vi "Teleop.vi"(10 "Match Info":T1={"Autonomous Elapsed Seconds"=0.0, "TeleOp Elapsed Seconds"=0.0, "Disabled Elapsed Seconds"=0.0, "Visited Autonomous"=FALSE, "Visited TeleOp"=FALSE, "Visited Disabled"=FALSE, "Autonomous Settings"={"Autonomous Style"=enum."Independent", "VI Refnum"=refnum}}, 11 "Call Context":T2) -> ()   [LabVIEW 2011]
doc: "This VI is called for each TeleOp packet received from the DS where the robot is not disabled. It is often used to read from the joysticks and update I/O or to update setpoints for timed control loops. It should complete and return within 20 milliseconds or it may miss DS packets."
uses:
  <vilib>/Rock Robotics/WPI/DriverStation/WPI_DriverStationDerivedRobotMode.ctl
  <vilib>/Rock Robotics/WPI/DriverStation/WPI_DriverStationMatch Info.ctl
  <vilib>/Rock Robotics/WPI/Relay/WPI_RelayValue.ctl
  Robot Global Data.vi
  Manual-Auto.vi
panel:
  out "shooter rpm":dbl
  out "Distance":dbl
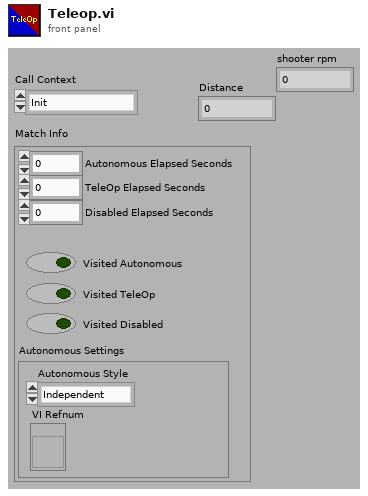
[diagram p1: front panel]
types:
  T1 = typedef "WPI_DriverStationMatch Info.ctl" = cluster{"Autonomous Elapsed Seconds":dbl, "TeleOp Elapsed Seconds":dbl, "Disabled Elapsed Seconds":dbl, "Visited Autonomous":bool, "Visited TeleOp":bool, "Visited Disabled":bool, "Autonomous Settings":cluster{"Autonomous Style":enum16{"Iterative", "Independent"}, "VI Refnum":refnum<vi>}}
  T2 = typedef "WPI_DriverStationDerivedRobotMode.ctl" = enum16{"Init", "Execute", "Stop"}
  T3 = typedef "WPI_RelayValue.ctl" = enum16{"Off", "On", "Forward", "Reverse"}
  T4 = typedef "WPI_EncoderDevRef.ctl" = cluster{"DevStatus":errorcluster, "EncoderIndex":T5, "CounterIndex":T6, "DistancePerCount":dbl, "Decoding Type":T7}
  T5 = typedef "FPGA_EncoderIdx.ctl" = enum8{"Enc 0", "Enc 1", "Enc 2", "Enc 3", "Invalid"}
  T6 = typedef "FPGA_CounterCtrSystemIndex.ctl" = enum8{"Ctr 0", "Ctr 1", "Ctr 2", "Ctr 3", "Ctr 4", "Ctr 5", "Ctr 6", "Ctr 7", "Invalid"}
  T7 = typedef "WPI_EncoderType.ctl" = enum16{"1x", "2x", "4x"}
  T8 = typedef "WPI_JoystickDevRef.ctl" = cluster{"Device":T9}
  T9 = typedef "WPI_JoystickDeviceEnum.ctl" = enum16{"USB 1", "USB 2", "USB 3", "USB 4", "Kinect 1", "Kinect 2"}
  T10 = typedef "WPI_JoystickButtonState.ctl" = cluster{"Button 1":bool, "Button 2":bool, "Button 3":bool, "Button 4":bool, "Button 5":bool, "Button 6":bool, "Button 7":bool, "Button 8":bool, "Button 9":bool, "Button 10":bool, "Button 11":bool, "Button 12":bool}
  T11 = cluster{"axis 1 (x)":dbl, "axis 2 (y)":dbl, "axis 3 (throttle)":dbl, "axis 4":dbl, "axis 5":dbl, "axis 6":dbl}
  T12 = typedef "WPI_RelayDevRef.ctl" = cluster{"DevStatus":errorcluster, "Relay Channel":T13, "Digital Module":T14, "Relay Direction":T15}
  T13 = typedef "FPGA_DIORelayChannel.ctl" = enum8{"Relay 1", "Relay 2", "Relay 3", "Relay 4", "Relay 5", "Relay 6", "Relay 7", "Relay 8", "Invalid"}
  T14 = typedef "FPGA_TypedefDigitalModule.ctl" = enum16{"Digital Module 1", "Digital Module 2"}
  T15 = typedef "WPI_RelayDirection.ctl" = enum16{"Both directions", "Forward only", "Reverse only"}
  T16 = typedef "WPI_DigitalInputDevRef.ctl" = cluster{"DevStatus":errorcluster, "DIO Channel":T17, "Digital Module":T14}
  T17 = typedef "FPGA_DIOChannel.ctl" = enum8{"DIO 1", "DIO 2", "DIO 3", "DIO 4", "DIO 5", "DIO 6", "DIO 7", "DIO 8", "DIO 9", "DIO 10", "DIO 11", "DIO 12", "DIO 13", "DIO 14", "Invalid"}
  T18 = typedef "WPI_RobotDriveDevRef.ctl" = cluster{"DevStatus":errorcluster, "Motors[]":T19[], "Square Inputs":bool, "Max Output":dbl, "Isochronous":bool}
  T19 = typedef "WPI_MotorControlDeviceRef.ctl" = cluster{"DeviceStatus":errorcluster, "Type":enum16{"PWM", "CAN"}, "PWM":cluster{"Digital Module":T14, "PWM Channel":T20, "DeadBand":T21}, "CAN":cluster{"Device Number":u8, "Control Mode":T22, "Semaphore":T23, "Max Vout":dbl}, "Invert":bool, "TransformRef":T24, "InvTransformRef":T24}
  T20 = typedef "FPGA_DIOPWMChannel.ctl" = enum8{"PWM 1", "PWM 2", "PWM 3", "PWM 4", "PWM 5", "PWM 6", "PWM 7", "PWM 8", "PWM 9", "PWM 10", "Invalid"}
  T21 = typedef "WPI_PWMDeadband.ctl" = cluster{"Name":string, "maxPositivePwm":i32, "minPositivePwm":i32, "centerPwm":i32, "maxNegativePwm":i32, "minNegativePwm":i32, "angularRange":u16}
  T22 = typedef "WPI_CANJaguar_ControlMode.ctl" = enum8{"Percent VBus", "Current", "Speed", "Position", "Voltage"}
  T23 = typedef "Semaphore RefNum" = refnum<k1>
  T24 = typedef "WPI_PWMTransform_ConPane.ctl" = refnum<vi>
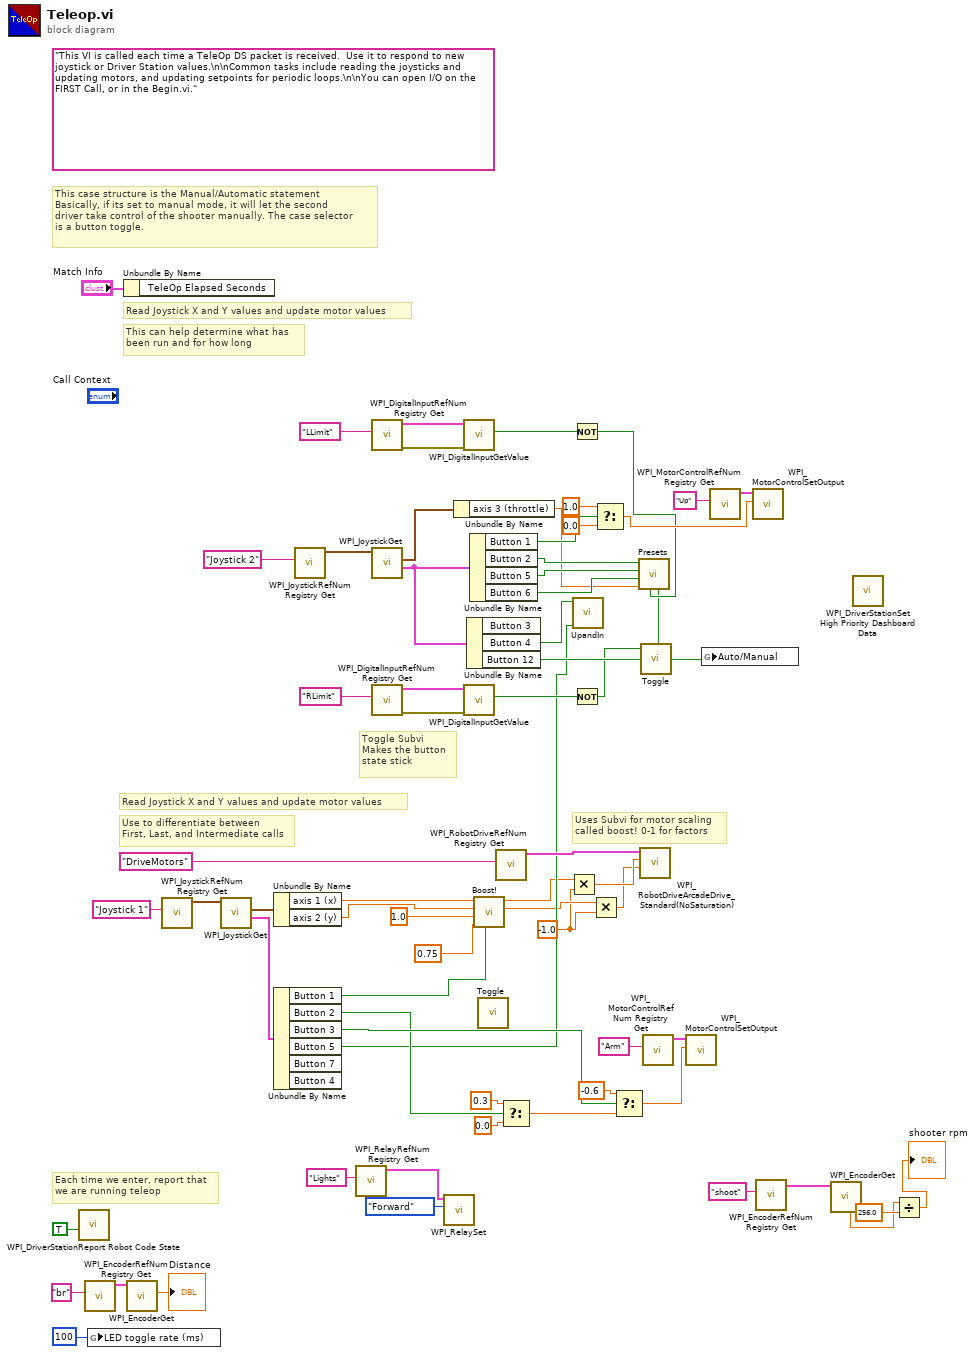
[diagram p0: block diagram]
diagram:
  w1 = -1.0 ("y")
  (unwired) "This VI is called each time a TeleOp DS packet is received.  Use it to respond to new joystick or Driver Station values.\n\nCommon tasks include reading the joysticks and updating motors, and updating setpoints for periodic loops.\n\nYou can open I/O on the FIRST Call, or in the Begin.vi."
  # "Toggle Subvi\nMakes the button\nstate stick"
  # "Uses Subvi for motor scaling\ncalled boost! 0-1 for factors"
  # "Read Joystick X and Y values and update motor values"
  # "This case structure is the Manual/Automatic statement\nBasically, if its set to manual mode, it will let the second \ndriver take control of the shooter manually. The case selector\nis a button toggle."
  # "Each time we enter, report that\nwe are running teleop"
  # "Use to differentiate between\nFirst, Last, and Intermediate calls"
  # "This can help determine what has\nbeen run and for how long"
  # "Read Joystick X and Y values and update motor values"
  n1 = call <vilib>:"WPI_DriverStationReport Robot Code State.vi"("TeleOp"=TRUE ("Autonomous")) -> ()  [unwired: 10 in, 1 out]
  n2 = call <vilib>:"WPI_EncoderRefNum Registry Get.vi"("refnum name"="br") -> ("EncoderDevRef"=w44:T4)  [unwired: 9 in, 1 out]
  n3 = global write "Robot Global Data.vi" "LED toggle rate (ms)"(u32 100 ("LED ms toggle rate")) -> ()
  n4 = Unbundle By Name("Match Info") -> ()  [unwired: 1 out]
  n5 = call <vilib>:"WPI_EncoderGet.vi"("EncoderDevRef"=w44) -> ("Distance"=→"Distance":dbl)  [unwired: 5 in, 5 out]
  n6 = call <vilib>:"WPI_JoystickRefNum Registry Get.vi"("refnum name"="Joystick 1") -> ("JoystickDevRef"=w60:T8)  [unwired: 1 in, 9 out]
  n7 = call <vilib>:"WPI_JoystickGet.vi"("JoystickDevRef"=w60) -> ("Buttons"=w59:T10, "Axes"=w62:T11)  [unwired: 1 in, 4 out]
  n8 = Unbundle By Name(w62) -> ("axis 1 (x)"=w41:dbl, "axis 2 (y)"=w40:dbl)
  n9 = Unbundle By Name(w59) -> ("Button 1"=w39:bool, "Button 2"=w30:bool, "Button 3"=w45:bool, "Button 5"=w29:bool)  [unwired: 2 out]
  n10 = call <vilib>:"WPI_JoystickRefNum Registry Get.vi"("refnum name"="Joystick 2") -> ("JoystickDevRef"=w56:T8)  [unwired: 1 in, 9 out]
  n11 = call <vilib>:"WPI_RelayRefNum Registry Get.vi"("refnum name"="Lights") -> ("RelayDevRef"=w9:T12)  [unwired: 9 in, 1 out]
  n12 = call <vilib>:"WPI_DigitalInputRefNum Registry Get.vi"("refnum name"="LLimit") -> ("error out"=w52:errorcluster, "DigitalInputDevRef"=w51:T16)  [unwired: 9 in]
  n13 = call <vilib>:"WPI_JoystickGet.vi"("JoystickDevRef"=w56) -> ("Buttons"=w47:T10, "Axes"=w58:T11)  [unwired: 1 in, 4 out]
  n14 = call <vilib>:"WPI_DigitalInputRefNum Registry Get.vi"("refnum name"="RLimit") -> ("error out"=w55:errorcluster, "DigitalInputDevRef"=w54:T16)  [unwired: 9 in]
  n15 = call <vilib>:"WPI_RelaySet.vi"("RelayValue"=WPI_RelayValue."Forward", "RelayDevRef"=w9) -> ()  [unwired: 8 in, 2 out]
  n16 = Unbundle By Name(w58) -> ("axis 3 (throttle)"=w19:dbl)
  n17 = call <vilib>:"WPI_DigitalInputGetValue.vi"("error in (no error)"=w52, "DigitalInputDevRef"=w51) -> ("Value"=w48:bool)  [unwired: 7 in, 2 out]
  n18 = call <vilib>:"WPI_DigitalInputGetValue.vi"("error in (no error)"=w55, "DigitalInputDevRef"=w54) -> ("Value"=w49:bool)  [unwired: 7 in, 2 out]
  n19 = Unbundle By Name(w47) -> ("Button 4"=w46:bool, "Button 12"=w38:bool)  [unwired: 1 out]
  n20 = Unbundle By Name(w47) -> ("Button 1"=w26:bool, "Button 2"=w22:bool, "Button 5"=w21:bool, "Button 6"=w20:bool)
  n21 = call "Boost!.vi"("Boost Ctrl"=w39, "Normal Factor"=0.75, "Boost Factor"=1.0, "Axis(y)"=w40, "Axis(x)"=w41) -> ("Motor Out(y)"=w2:dbl, "Motor Out(x)"=w5:dbl)  [unwired: 5 in]
  n22 = call "Toggle.vi"() -> ()  [unwired: 1 in, 1 out]
  n23 = call <vilib>:"WPI_RobotDriveRefNum Registry Get.vi"("refnum name"="DriveMotors") -> ("RobotDriveDevRef"=w63:T18)  [unwired: 1 in, 9 out]
  n24 = Select(t=0.3, s=w30, f=0.0) -> (s? t:f=w33:dbl)
  n25 = Multiply(x=w5, y=w1) -> (x*y=w4:dbl)
  n26 = Not(x=w48) -> (.not. x?=w18:bool)
  n27 = Not(x=w49) -> (.not. x?=w17:bool)
  n28 = call "UpandIn.vi"("Out"=w46, "In"=w29) -> ()  [unwired: 9 in]
  n29 = Multiply(x=w2, y=w1) -> (x*y=w3:dbl)
  n30 = Select(t=1.0, s=w26, f=0.0) -> (s? t:f=w25:dbl)
  n31 = Select(t=-0.6, s=w45, f=w33) -> (s? t:f=w31:dbl)
  n32 = call "Presets.vi"("RLimit"=w17, "LLimit"=w18, "TwistAxis"=w19, "Key"=w20, "STOP"=w21, "100"=w22) -> ()  [unwired: 6 in]
  n33 = call <vilib>:"WPI_RobotDriveArcadeDrive_Standard(NoSaturation).vi"("Y axis value"=w3, "X axis value"=w4, "RobotDriveDevRef"=w63) -> ()  [unwired: 1 in, 8 out]
  n34 = call "Toggle.vi"("Boolean"=w38) -> ("Boolean 2"=w11:bool)
  n35 = call <vilib>:"WPI_MotorControlRefNum Registry Get.vi"("refnum name"="Arm") -> ("MotorControlDevRef"=w35:T19)  [unwired: 9 in, 1 out]
  n36 = call <vilib>:"WPI_MotorControlSetOutput.vi"("Output"=w31, "MotorControlDevRef"=w35) -> ()  [unwired: 8 in, 2 out]
  n37 = global write "Manual-Auto.vi" "Auto/Manual"(w11) -> ()
  n38 = call <vilib>:"WPI_MotorControlRefNum Registry Get.vi"("refnum name"="Up") -> ("MotorControlDevRef"=w28:T19)  [unwired: 9 in, 1 out]
  n39 = call <vilib>:"WPI_MotorControlSetOutput.vi"("Output"=w25, "MotorControlDevRef"=w28) -> ()  [unwired: 8 in, 2 out]
  n40 = call <vilib>:"WPI_EncoderRefNum Registry Get.vi"("refnum name"="shoot") -> ("EncoderDevRef"=w16:T4)  [unwired: 9 in, 1 out]
  n41 = call <vilib>:"WPI_EncoderGet.vi"("EncoderDevRef"=w16) -> ("Rate"=w12:dbl)  [unwired: 5 in, 5 out]
  n42 = call <vilib>:"WPI_DriverStationSet High Priority Dashboard Data.vi"() -> ()  [unwired: 11 in, 1 out]
  n43 = Divide(x=w12, y=256.0) -> (x/y=→"shooter rpm":dbl)
